vi "VI Server_SetCursor_BUSY.vi"(8 "error in":errorcluster, 11 "VI Server.RefsCluster":T1) -> (0 "error out":errorcluster, 3 "VI Server.RefsCluster.DUP":T1)   [LabVIEW 2020]
uses:
  VI Server_TypeDefs/VI Server_RefsCluster.ctl
  <vilib>/Utility/cursorutil.llb/Set Cursor (Icon Pict).vi
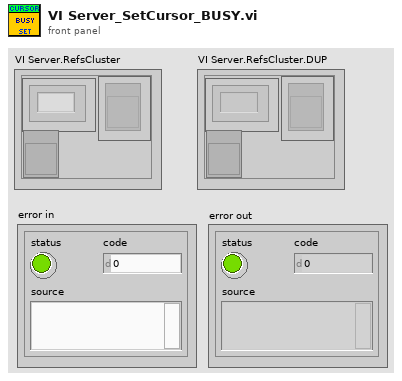
[diagram p1: front panel]
types:
  T1 = typedef "VI Server_RefsCluster.ctl" = cluster{"Labels":string[], "Refs":refnum<vi>[], "VI Ref":refnum<vi>}
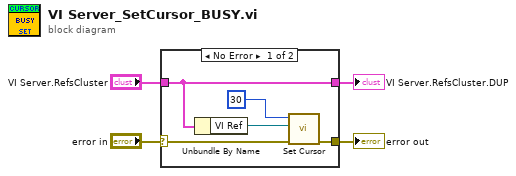
[diagram p0: block diagram]
diagram:
  n1 = case shown="No Error" "error in" {
    selector: "error in" -> [w6 w10]
    tunnel: [w8 w10] -> w4
    tunnel: "VI Server.RefsCluster" -> [w5 _]
    tunnel: [w5 _] -> w1
    frame No Error {
      n2 = Unbundle By Name(w5) -> ("VI Ref"=w7:refnum<vi>)
      n3 = call-poly <vilib>:"Set Cursor.vi"("error in (no error)"=w6, "VI reference (current VI)"=w7, "icon"=u16 30) -> ("error out"=w8:errorcluster)  [unwired: 7 in, 1 out]
    }
    frame Error {
    }
  }
  "VI Server.RefsCluster.DUP" <- w1
  "error out" <- w4
